vi "HSE_AboutScreen.vi"() -> ()   [LabVIEW 2022 SP3, in "hse-ui.lvlib"]
doc: "____\nHAMPEL SOFTWARE ENGINEERING v3.8.0 (2023-12-18 14:41)"
uses:
  hse-ui.lvlib
  hse-misc/Event/Event_GenericReference.ctl
  hse-misc/Event/Event_GenericDatatype.ctl
  <vilib>/Utility/cursorutil.llb/Set Cursor (Icon Pict).vi
  <vilib>/Platform/browser.llb/Open URL in Default Browser (string).vi
  hse-misc/hse-misc.lvlib
panel:
  in  "Btn_Website":bool
  in  "Btn_Close":bool
  out "String":string
  out "Slide":u8(slide) scale=0.0..100.0
  in  "Splash VI Event":T1
  # "HAMPEL SOFTWARE ENGINEERING\nBürgerbräu, Geb. 13 (Picherei)\nFrankfurter Straße 87\n97082 Würzburg, Germany"
  # "T: +49 931 78023687\nF: +49 931 78023688\noffice@hampel-soft.com\nwww.hampel-soft.com"
  # "...visit us on"
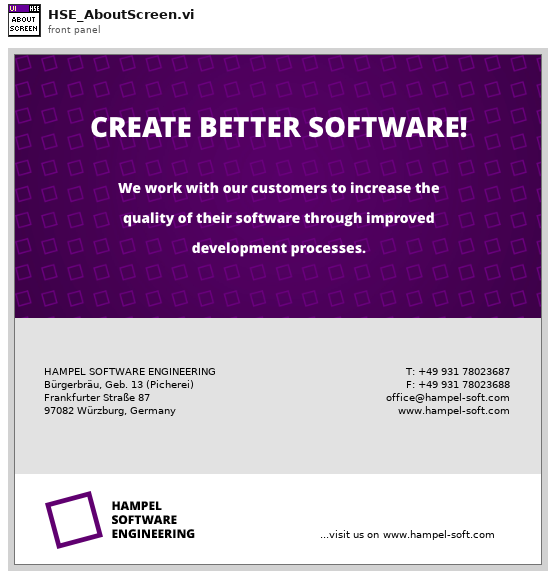
[diagram p1: front panel]
types:
  T1 = typedef "hse-misc.lvlib/Event_GenericReference.ctl" = refnum<user-event>
  T2 = enum32{"Invalid", "Standard", "Closed", "Hidden", "Minimized", "Maximized"}
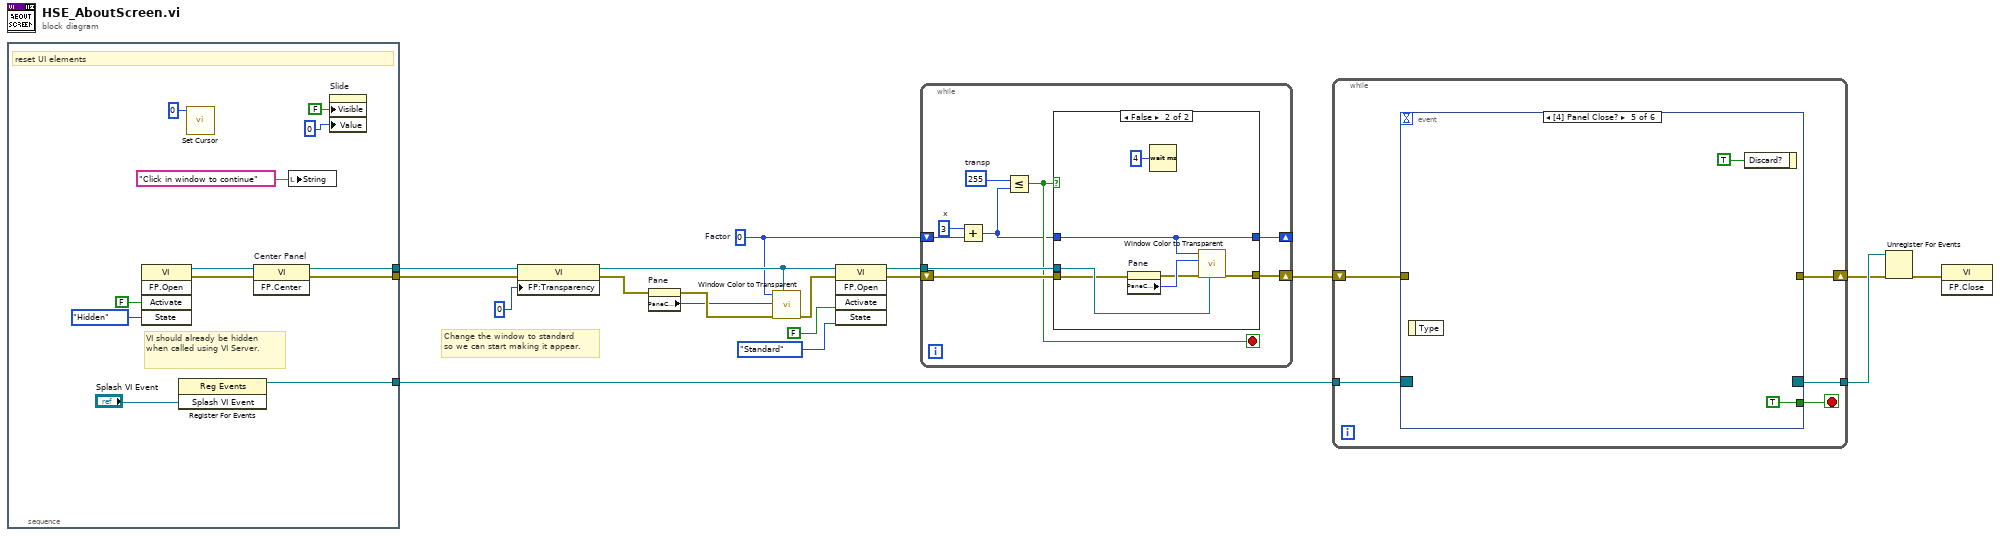
[diagram p0: block diagram]
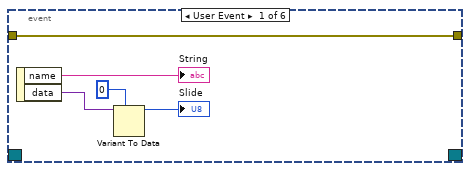
[diagram p3: hidden frame]
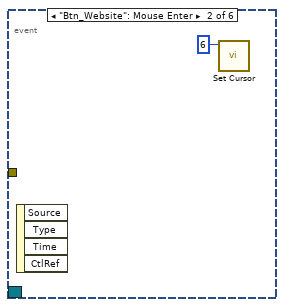
[diagram p4: hidden frame]
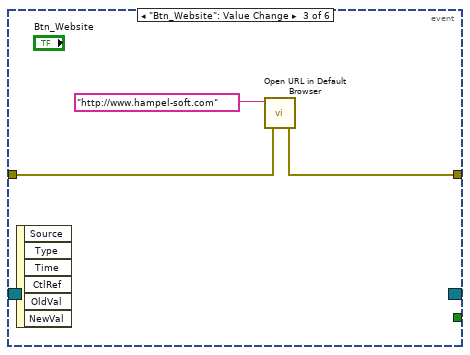
[diagram p5: hidden frame]
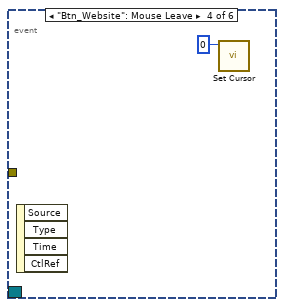
[diagram p6: hidden frame]
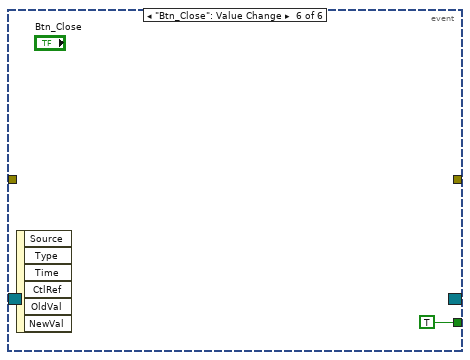
[diagram p7: hidden frame]
diagram:
  w3 = u8 0  # Factor
  # "Change the window to standard\nso we can start making it appear."
  n1 = stacked-sequence {
    tunnel: [w24] -> w15
    tunnel: [w23] -> w14
    tunnel: [w27] -> w16
    frame #0 {
      # "VI should already be hidden when called using VI Server."
      # "reset UI elements"
      n2 = invoke class="VI" method="FP.Open"("Activate"=FALSE ("Activate?"), "State"=T2."Hidden") -> (reference out=w25:refnum<vi>, error out=w26:errorcluster)  [unwired: 3 in, 3 out]
      n3 = register-events("Splash VI Event") -> (reference out=w27:refnum<event-registration>)  [unwired: 2 in, 1 out]
      n4 = call-poly <vilib>:"Set Cursor.vi"("icon"=u16 0) -> ()  [unwired: 9 in, 2 out]
      n5 = invoke on="Center Panel" class="VI" method="FP.Center"(reference=w25, error in=w26) -> (reference out=w24:refnum<vi>, error out=w23:errorcluster)  [unwired: 1 in, 1 out]
      n6 = local write "String"("Click in window to continue") -> ()
      n7 = property on="Slide" class="Slide (strict)"("Visible"=FALSE, "Value"=u8 0 ("Slide")) -> ()  [unwired: 2 in, 2 out]
    }
  }
  n8 = property class="VI"(reference=w15, error in=w14, "FP:Transparency"=u8 0 ("t")) -> (reference out=w5:refnum<vi>, error out=w7:errorcluster)
  n9 = property on="Pane" class="Pane"(error in=w7) -> (error out=w11:errorcluster, "PaneColor"=w10:u32)  [unwired: 1 in, 1 out]
  n10 = call "Window Color to Transparent.vi"("Calling VI's reference"=w5, "error in (no error)"=w11, "Color to Replace"=w10, "Factor"=w3) -> ("error out"=w6:errorcluster)  [unwired: 7 in]
  n11 = invoke class="VI" method="FP.Open"(reference=w5, error in=w6, "Activate"=FALSE ("Activate?"), "State"=T2."Standard") -> (reference out=w9:refnum<vi>, error out=w8:errorcluster)  [unwired: 1 in, 3 out]
  n12 = while {
    shift-right: [w37] -> _
    shift-left: w3 -> [w33]
    shift-right: [w36] -> w17
    shift-left: w8 -> [w35]
    tunnel: w9 -> [w38]
    stop <- w34 stop-if-true
    w31 = u8 3  # x
    w39 = u8 255  # transp
    n13 = Add(x=w31, y=w33) -> (x+y=w32:u8)
    n14 = Less Or Equal?(x=w39, y=w32) -> (x <= y?=w34:bool)
    n15 = case shown="False" w34 {
      tunnel: w32 -> [w41 w45]
      tunnel: w38 -> [_ w46]
      tunnel: [w41 w45] -> w37
      tunnel: [w40 w44] -> w36
      tunnel: w35 -> [w40 w43]
      frame True {
      }
      frame False {
        n16 = property on="Pane" class="Pane"(error in=w43) -> (error out=w47:errorcluster, "PaneColor"=w48:u32)  [unwired: 1 in, 1 out]
        n17 = Wait (ms)(milliseconds to wait=u32 4) -> ()  [unwired: 1 out]
        n18 = call "Window Color to Transparent.vi"("Calling VI's reference"=w46, "error in (no error)"=w47, "Color to Replace"=w48, "Factor"=w45) -> ("error out"=w44:errorcluster)  [unwired: 7 in]
      }
    }
  }
  n19 = while {
    shift-right: [w53] -> w2
    shift-left: w17 -> [w51]
    tunnel: [w50] -> w18
    tunnel: w16 -> [w49]
    stop <- w52 stop-if-true
    n20 = event shown="[4] Panel Close?" {
      selector: w49 -> [_ _ _ _ _ _]
      dyn-events: [_ _ _ _ _ _] -> w50
      timeout: _ -> [_ _ _ _ _ _]
      tunnel: w51 -> [w58 _ w60 _ _ _]
      tunnel: [w58 _ w61 _ _ _] -> w53
      tunnel: [_ _ _ _ TRUE ("Close") TRUE ("Close")] -> w52
      event User Event {
        n21 = event-data() -> ("name"=→"String":string, "data"=w57:variant)  [unwired: 1 in]
        n22 = Variant To Data(type=u8 0 ("Slide"), Variant=w57) -> (data=→"Slide":u8)  [unwired: 1 in, 1 out]
      }
      event "Btn_Website": Mouse Enter {
        n23 = event-data() -> ()  [unwired: 1 in, 4 out]
        n24 = call-poly <vilib>:"Set Cursor.vi"("icon"=u16 6) -> ()  [unwired: 9 in, 2 out]
      }
      event "Btn_Website": Value Change {
        n25 = event-data() -> ()  [unwired: 1 in, 6 out]
        n26 = call-poly <vilib>:"Open URL in Default Browser.vi"("error in (no error)"=w60, "URL"="http://www.hampel-soft.com" ("Link")) -> ("error out"=w61:errorcluster)  [unwired: 4 in, 1 out]
      }
      event "Btn_Website": Mouse Leave {
        n27 = event-data() -> ()  [unwired: 1 in, 4 out]
        n28 = call-poly <vilib>:"Set Cursor.vi"("icon"=u16 0) -> ()  [unwired: 9 in, 2 out]
      }
      event Panel Close? {
        n29 = event-data() -> ()  [unwired: 1 in, 1 out]
        n30 = event-data("Discard?"=TRUE) -> ()  [unwired: 1 in, 1 out]
      }
      event "Btn_Close": Value Change {
        n31 = event-data() -> ()  [unwired: 1 in, 6 out]
      }
    }
  }
  n32 = Unregister For Events(event registration refnum=w18, error in=w2) -> (error out=w1:errorcluster)
  n33 = invoke class="VI" method="FP.Close"(error in=w1) -> ()  [unwired: 2 in, 3 out]
